vi "SearchNode.vi"(8 "error in (no error)":errorcluster, 10 "GraphNode in":refnum<data-value>, 11 "GraphSearch in":refnum<class "GraphSearch.lvclass">) -> (0 "error out":errorcluster, 1 "found":bool, 2 "GraphNode out":refnum<data-value>, 3 "GraphSearch out":refnum<class "GraphSearch.lvclass">)   [LabVIEW 2009, in "GraphSearch.lvclass"]
uses:
  GraphSearch.lvclass
  GraphNode/GraphNode.lvclass
  Node/Node.lvclass
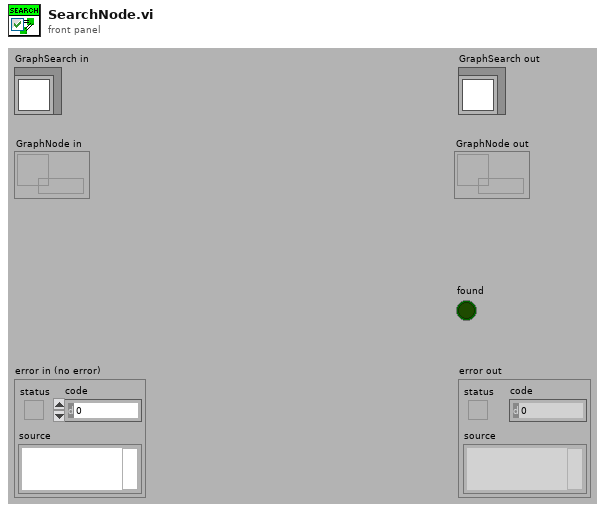
[diagram p1: front panel]
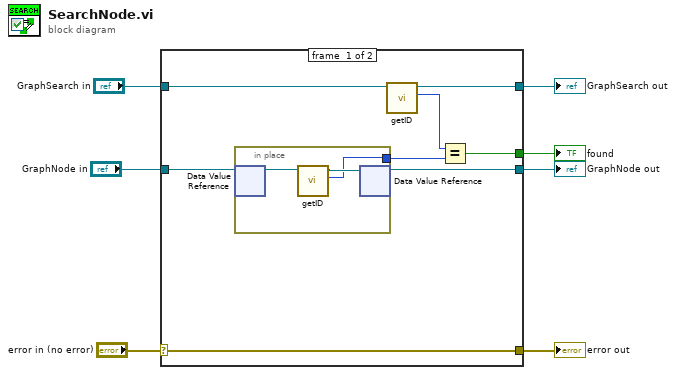
[diagram p0: block diagram]
diagram:
  n1 = case shown="No Error" "error in (no error)" {
    selector: "error in (no error)" -> [w15 w21]
    tunnel: [w15 w21] -> w6
    tunnel: [w12 w20] -> w4
    tunnel: "GraphSearch in" -> [w13 w20]
    tunnel: "GraphNode in" -> [w14 w19]
    tunnel: [w9 w19] -> w2
    tunnel: [w8 _] -> w1
    frame #0 {
      n2 = in-place {
        in-place-border: [w16] -> w11
        n3 = in-place-dvr #1(w14) -> (w18:refnum<class "GraphNode.lvclass">)  [unwired: 1 out]
        n4 = call "getID.vi"("Node in"=w18) -> ("ID"=w16:u32, "Node out"=w17:refnum<class "GraphNode.lvclass">)  [unwired: 8 in, 1 out]
        n5 = in-place-dvr #1(w17) -> (w9:refnum<data-value>)  [unwired: 1 out]
      }
      n6 = call "getID.vi"("GraphSearch in"=w13) -> ("ID"=w10:u32, "GraphSearch out"=w12:refnum<class "GraphSearch.lvclass">)  [unwired: 8 in, 1 out]
      n7 = Equal?(x=w10, y=w11) -> (x = y?=w8:bool)
    }
    frame #1 {
    }
  }
  "error out" <- w6
  "GraphSearch out" <- w4
  "GraphNode out" <- w2
  "found" <- w1
